vi "SendRequestApproval.vi"(8 "error in (no error)":errorcluster, 10 "calibration-id":i32, 11 "ByteGSAPIBase in":refnum<class "ByteQXAPIBase.lvclass">) -> (0 "error out":errorcluster, 2 "controls":T1(array[cluster]), 3 "ByteGSAPIBase out":refnum<class "ByteQXAPIBase.lvclass">)   [LabVIEW 2019, in "ByteQXWebAPI.lvlib" / "ByteQXAPIBase.lvclass"]
doc: "Send the approal request based on the calibration-id"
uses:
  ByteQXAPIBase.lvclass
  <vilib>/Bytelabs/ByteREST/ByteRESTClass/ByteRESTBase/HTTP/Status_Code.ctl
  RequestApproval.ctl
  Private/module.ctl
  ByteQXAPIBase.lvclass/ByteQXAPIBase.ctl
  <vilib>/Bytelabs/ByteREST/ByteRESTClass/ByteRESTBase/RESTBase.lvclass
panel:
  in  "send notification":bool
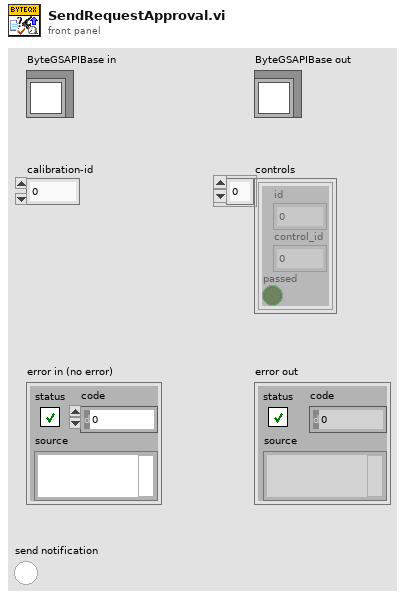
[diagram p1: front panel]
types:
  T1 = cluster{"id":u32, "control_id":u32, "passed":bool}[]
  T2 = typedef "ByteQXWebAPI.lvlib/ByteQXAPIBase.lvclass/module.ctl" = enum16{"gs", "tms"}
  T3 = typedef "ByteQXWebAPI.lvlib/ByteQXAPIBase.lvclass/RequestApproval.ctl" = cluster{"controls":cluster{"id":u32, "control_id":u32, "passed":bool}[]}
  T4 = cluster{"calibration_id":i32, "notification_active":bool}
  T5 = typedef "ByteREST.lvlib/RESTBase.lvclass/Status_Code.ctl" = u16
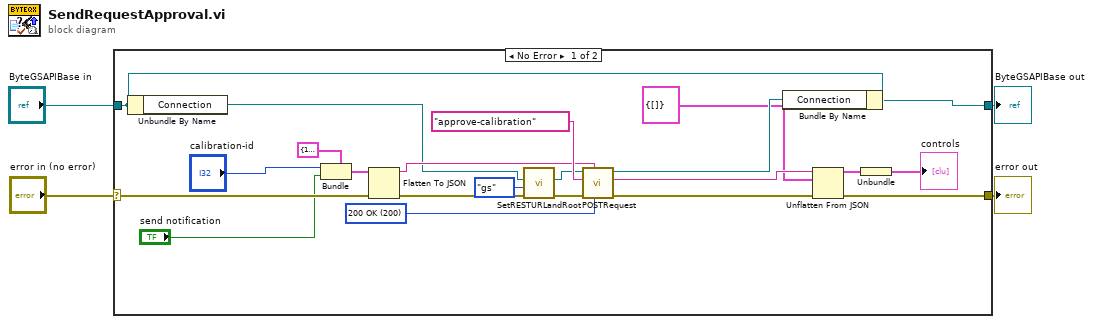
[diagram p0: block diagram]
diagram:
  n1 = case shown="No Error" "error in (no error)" {
    selector: "error in (no error)" -> [w22 w28]
    tunnel: [w17 w28] -> w3
    tunnel: [w25 w27] -> w1
    tunnel: "ByteGSAPIBase in" -> [w26 w27]
    frame No Error {
      w19 = T5 200 items=["200 OK"=200, "201 Created"=201, "400 Bad Request"=400, "401 Unauthorized"=401, "403 Forbidden"=403, "404 Not Found"=404, "405 Method Not Allowed"=405, "406 Not Acceptable"=406, "500 Internal Server Error"=500] ("expected response")
      n2 = Unbundle By Name(w26) -> ("Connection"=w7:refnum<class "RESTBase.lvclass">)
      n3 = Bundle(cluster=T4 {"calibration_id"=1234, "notification_active"=FALSE}, "calibration_id"="calibration-id", "notification_active"="send notification") -> (w14:T4)
      n4 = Flatten To JSON(anything=w14, error in (no error)=w22) -> (JSON string=w18:string, 11:w9:errorcluster)  [unwired: 1 in]
      n5 = call "SetRESTURLandRoot.vi"("error in (no error)"=w9, "module"=module."gs", "ByteREST in"=w7) -> ("error out"=w8:errorcluster, "ByteREST out"=w6:refnum<class "RESTBase.lvclass">)  [unwired: 7 in]
      n6 = call-dynamic "POSTRequest.vi"("expected response"=w19, "Body in"=w18, "error in (no error)"=w8, "Request"="approve-calibration", "ByteRESTBase in"=w6) -> ("error out"=w20:errorcluster, "Body"=w21:string, "ByteRESTBase out"=w24:refnum<class "RESTBase.lvclass">)  [unwired: 3 in, 1 out]
      n7 = Bundle By Name(cluster=w26, "Connection"=w24) -> (w25:refnum<class "ByteQXAPIBase.lvclass">)
      n8 = Unflatten From JSON(JSON string=w21, type and defaults=T3 {"controls"=[]}, error in (no error)=w20) -> (value=w12:T3, error out=w17:errorcluster)  [unwired: 4 in]
      n9 = Unbundle(w12) -> ("controls"=→"controls":T1)
    }
    frame Error {
    }
  }
  "error out" <- w3
  "ByteGSAPIBase out" <- w1
